vi "AO gen.vi"(0 "X pixel":i32=512, 1 "X step (um)":dbl=0.1, 2 "Y step (um)":dbl=0.1, 3 "Y line":i32=512, 4 "error in":errorcluster) -> (5 "waveform output":waveform(dbl)[](array[waveform]), 7 "error out":errorcluster)   [LabVIEW 2012]
uses:
  <vilib>/Waveform/WDTOps.llb/WDT Append Waveforms DBL.vi
  <vilib>/measure/NI_MABase.lvlib
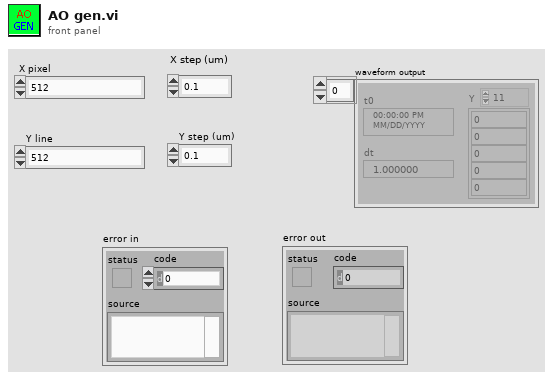
[diagram p1: front panel]
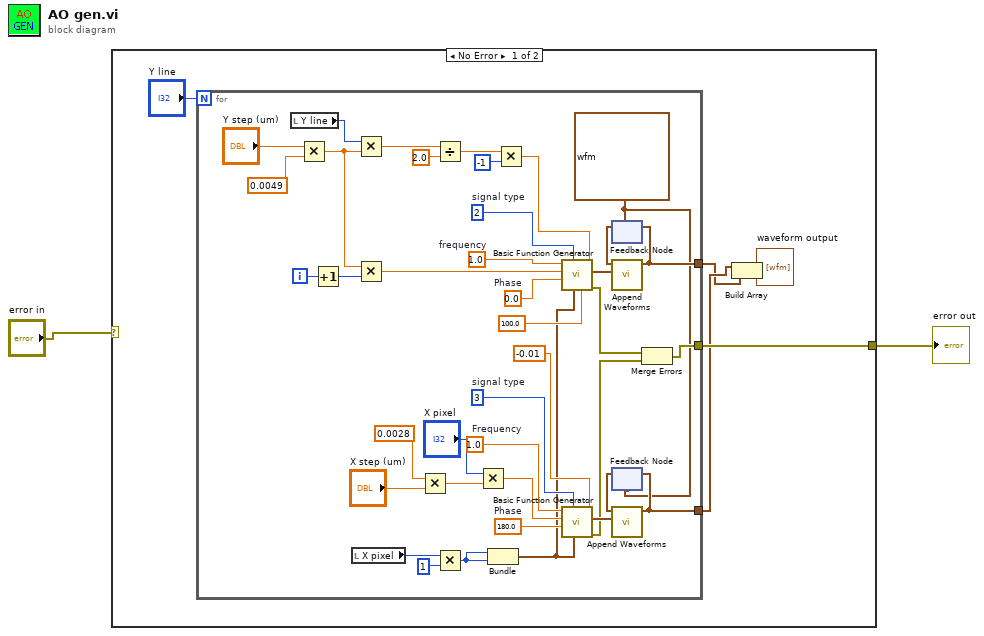
[diagram p0: block diagram]
diagram:
  n1 = case shown="No Error" "error in" {
    selector: "error in" -> [_ w47]
    tunnel: [w5 w47] -> w1
    frame No Error {
      n2 = for {
        N: "Y line" -> [_]
        tunnel: [w32] -> w3
        tunnel: [w37] -> w4
        tunnel: [w9] -> w5
        i -> [w35]
        w8 = waveform(dbl) {"t0"=timestamp(0 s since 1904-01-01), "dt"=1.0, "Y"=[]} ("waveform out")
        w36 = 0.0  # Phase
        w38 = 180.0  # Phase
        w41 = 3  # signal type
        w42 = 1.0  # Frequency
        w45 = 1.0  # frequency
        w44 = 2  # signal type
        n3 = local read "Y line"() -> (w16:i32)
        n4 = Multiply(x="Y step (um)", y=0.0049) -> (x*y=w17:dbl)
        n5 = Increment(x=w35) -> (x+1=w34:i32)
        n6 = local read "X pixel"() -> (w20:i32)
        n7 = Multiply(x=w16, y=w17) -> (x*y=w13:dbl)
        n8 = Multiply(x=w17, y=w34) -> (x*y=w19:dbl)
        n9 = Multiply(x=0.0028, y="X step (um)") -> (x*y=w22:dbl)
        n10 = Divide(x=w13, y=2.0) -> (x/y=w14:dbl)
        n11 = Multiply(x=w20, y=1) -> (x*y=w29:i32)
        n12 = Multiply(x="X pixel", y=w22) -> (x*y=w30:dbl)
        n13 = Bundle(w29, w29) -> (w27:cluster{i32, i32})  [unwired: 1 out]
        n14 = Multiply(x=w14, y=-1) -> (x*y=w15:dbl)
        n15 = call <vilib>:"Basic Function Generator.vi"("offset"=w15, "square wave duty cycle (%)"=100.0 ("duty cycle (%)"), "sampling info"=w27, "signal type"=w44, "phase"=w36, "amplitude"=w19, "frequency"=w45) -> ("error out"=w11:errorcluster, "signal out"=w43:waveform(dbl))  [unwired: 2 in, 1 out]
        n16 = call <vilib>:"Basic Function Generator.vi"("offset"=-0.01, "sampling info"=w27, "signal type"=w41, "phase"=w38, "amplitude"=w30, "frequency"=w42) -> ("error out"=w10:errorcluster, "signal out"=w39:waveform(dbl))  [unwired: 3 in, 1 out]
        n17 = feedback #1(w8) -> (w33:waveform(dbl))
        n18 = call-poly <vilib>:"Append Waveforms.vi"("waveform B"=w43, "waveform A"=w33) -> ("waveform out"=w32:waveform(dbl))  [unwired: 1 in, 8 out]
        n19 = feedback-in #1(w32) -> ()
        n20 = feedback #2(w8) -> (w40:waveform(dbl))
        n21 = call-poly <vilib>:"Append Waveforms.vi"("waveform B"=w39, "waveform A"=w40) -> ("waveform out"=w37:waveform(dbl))  [unwired: 1 in, 8 out]
        n22 = feedback-in #2(w37) -> ()
        n23 = Merge Errors(w11, w10) -> (w9:errorcluster)
      }
      n24 = Build Array ("创建数组")(w4, w3) -> (→"waveform output":waveform(dbl)[])
    }
    frame Error {
    }
  }
  "error out" <- w1
